vi "ELVIS III v1.0 AI Block Read.vi"(6 "AI FIFO Sample Rate":dbl=1000.0 min=1000.0 max=1000000.0, 7 "Scale Constants Array":T1, 8 "error in (no error)":errorcluster, 9 "Number of Samples":u32=1000, 10 "AI (N Samples) Channels List":T3, 11 "myRIO Ref In":T5) -> (0 "error out":errorcluster, 2 "dbl Scaled Value List":dbl[][](array[numeric]), 3 "myRIO Ref Out":T5)   [LabVIEW 2021]
uses:
  <vilib>/myRIO/Common/Instrument Driver Framework/Utilities/typedefs/myRIO v1.0 Reference.ctl
  <vilib>/myRIO/Common/Instrument Driver Framework/Utilities/typedefs/Generic FPGA Reference.ctl
  <vilib>/myRIO/Common/Instrument Driver Framework/myRIO v1.0/AI Block/typedefs/AI Block Channels List.ctl
  <vilib>/myRIO/Common/Instrument Driver Framework/myRIO v1.0/AI Block/typedefs/AI Block Channels Enum.ctl
  <vilib>/myRIO/Common/Instrument Driver Framework/Utilities/typedefs/Analog Scaling Constants List.ctl
  <vilib>/myRIO/Common/Instrument Driver Framework/Utilities/typedefs/Analog Scaling Constants.ctl
  <vilib>/myRIO/Common/Instrument Driver Framework/ELVIS III v1.0/AI Block/typedefs/ELVIS III AI Block Channels FPGA Reference.ctl
  <vilib>/myRIO/Common/Instrument Driver Framework/myRIO v1.0/Resource Manager/vis/myRIO v1.0 Block Write Configuration.vi
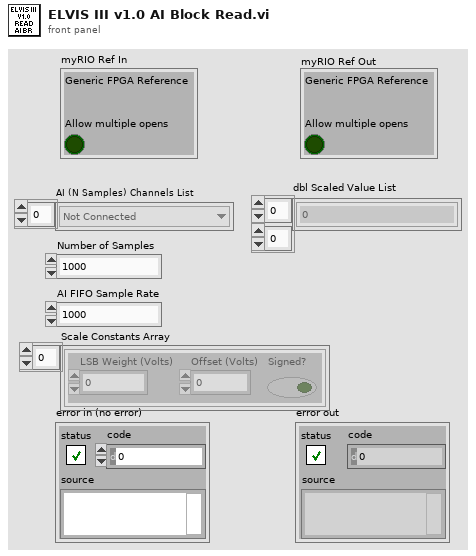
[diagram p1: front panel]
types:
  T1 = typedef "Analog Scaling Constants List.ctl" = T2[]
  T2 = typedef "Analog Scaling Constants.ctl" = cluster{"LSB Weight (Volts)":dbl, "Offset (Volts)":dbl, "Signed?":bool}
  T3 = typedef "AI Block Channels List.ctl" = T4[]
  T4 = typedef "AI Block Channels Enum.ctl" = enum16{"Not Connected", "A/AI0 (N Samples)", "A/AI1 (N Samples)", "A/AI2 (N Samples)", "A/AI3 (N Samples)", "A/AI4 (N Samples)", "A/AI5 (N Samples)", "A/AI6 (N Samples)", "A/AI7 (N Samples)", "A/AI0 (DIFF N Samples)", "A/AI1 (DIFF N Samples)", "A/AI2 (DIFF N Samples)", "A/AI3 (DIFF N Samples)", "B/AI0 (N Samples)", "B/AI1 (N Samples)", "B/AI2 (N Samples)", "B/AI3 (N Samples)", "B/AI4 (N Samples)", "B/AI5 (N Samples)", "B/AI6 (N Samples)", "B/AI7 (N Samples)", "B/AI0 (DIFF N Samples)", "B/AI1 (DIFF N Samples)", "B/AI2 (DIFF N Samples)", "B/AI3 (DIFF N Samples)"}
  T5 = typedef "myRIO v1.0 Reference.ctl" = cluster{"Generic FPGA Reference":T6, "Allow multiple opens":bool}
  T6 = typedef "Generic FPGA Reference.ctl" = refnum<k20>
  T7 = typedef "ELVIS III AI Block Channels FPGA Reference.ctl" = refnum<k20>
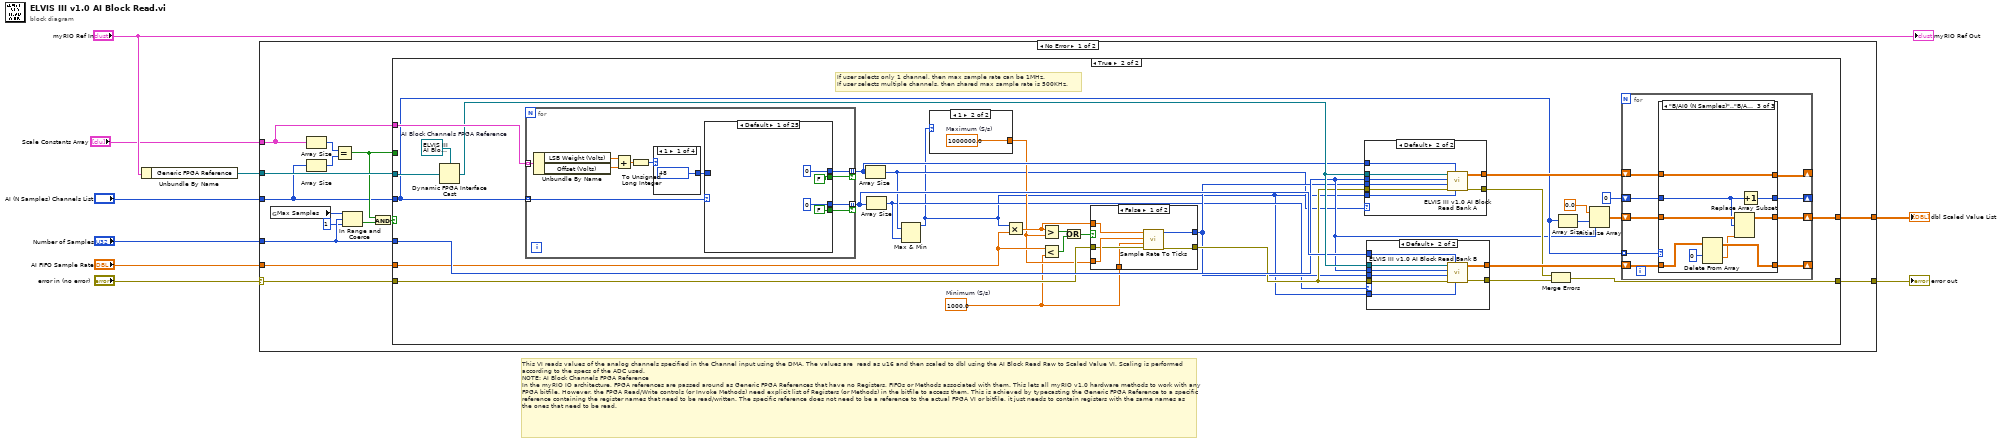
[diagram p0: block diagram]
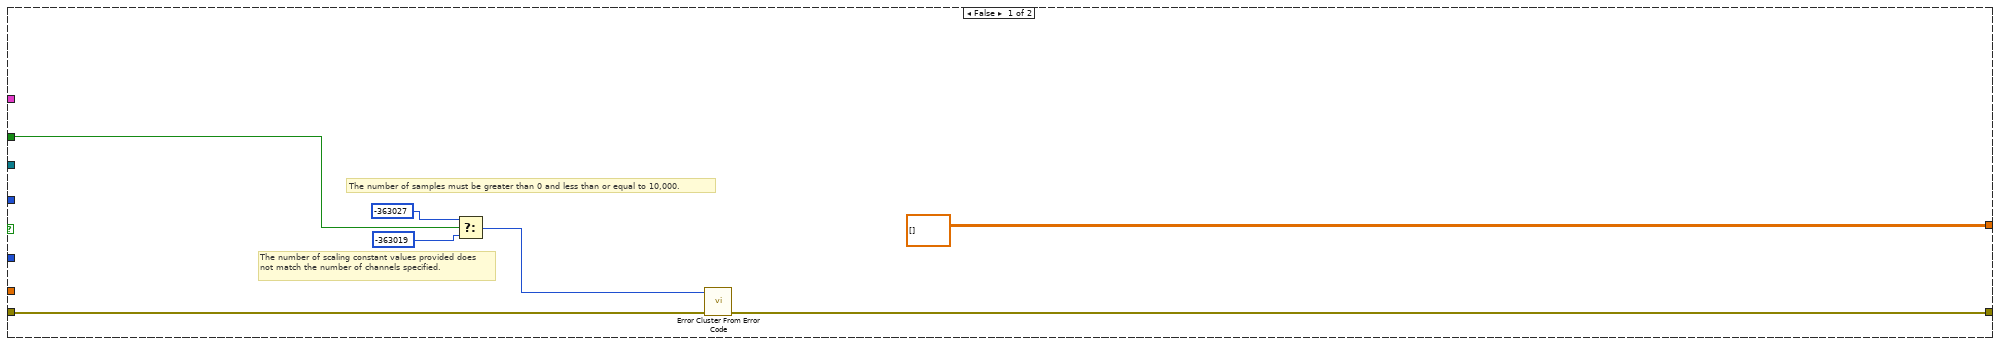
[diagram p2: hidden frame]
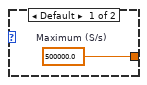
[diagram p3: hidden frame]
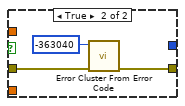
[diagram p4: hidden frame]
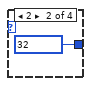
[diagram p5: hidden frame]
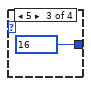
[diagram p6: hidden frame]
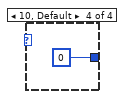
[diagram p7: hidden frame]
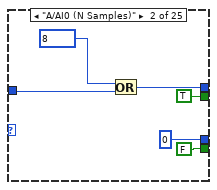
[diagram p8: hidden frame]
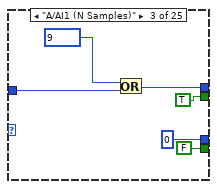
[diagram p9: hidden frame]
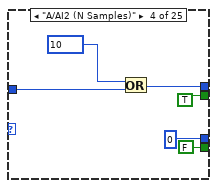
[diagram p10: hidden frame]
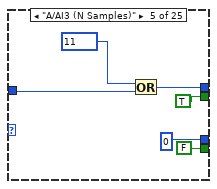
[diagram p11: hidden frame]
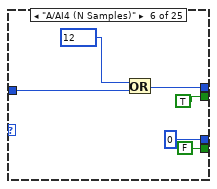
[diagram p12: hidden frame]
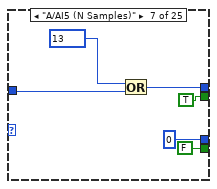
[diagram p13: hidden frame]
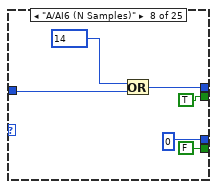
[diagram p14: hidden frame]
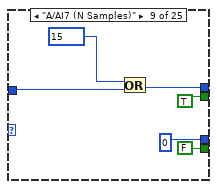
[diagram p15: hidden frame]
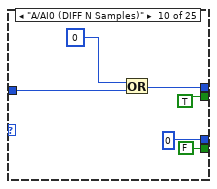
[diagram p16: hidden frame]
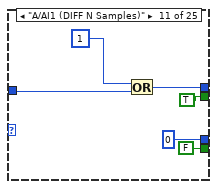
[diagram p17: hidden frame]
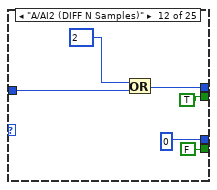
[diagram p18: hidden frame]
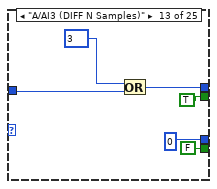
[diagram p19: hidden frame]
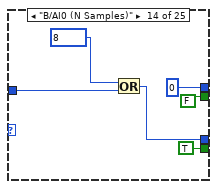
[diagram p20: hidden frame]
diagram:
  # "This VI reads values of the analog channels specified in the Channel input using the DMA. The values are  read as u16 and then scaled to dbl using the AI Block Read Raw to Scaled Value VI. Scaling is performed according to the specs of the ADC used.\nNOTE: AI Block Channels FPGA Reference\nIn the myRIO IO architecture, FPGA references are passed around as Generic FPGA References that have no Registers, FIFOs or Methods associated with them. This lets all myRIO v1.0 hardware methods to work with any FPGA bitfile. However, the FPGA Read/Write controls (or Invoke Methods) need explicit list of Registers (or Methods) in the bitfile to access them. This is achieved by typecasting the Generic FPGA Reference to a specific reference containing the register names that need to be read/written. The specific reference does not need to be a reference to the actual FPGA VI or bitfile, it just needs to contain registers with the same names as the ones that need to be read."
  n1 = Unbundle By Name("myRIO Ref In") -> ("Generic FPGA Reference"=w6:T6)
  n2 = case shown="No Error" "error in (no error)" {
    selector: "error in (no error)" -> [w10 w289]
    tunnel: w6 -> [w24 _]
    tunnel: [w23 w289] -> w9
    tunnel: [w22 dbl[][] [] ("dbl Scaled Value")] -> w8
    tunnel: "AI (N Samples) Channels List" -> [w12 _]
    tunnel: "AI FIFO Sample Rate" -> [w11 _]
    tunnel: "Number of Samples" -> [w16 _]
    tunnel: "Scale Constants Array" -> [w13 _]
    frame No Error {
      n3 = global read "myRIO v1.0 Block Write Configuration.vi" "Max Samples"() -> (w17:u32)
      n4 = Array Size(array=w13) -> (size(s)=w20:i32)
      n5 = Array Size(array=w12) -> (size(s)=w21:i32)
      n6 = Equal?(x=w20, y=w21) -> (x = y?=w18:bool)
      n7 = In Range and Coerce(upper limit=w17, x=w16, lower limit=u32 1) -> (In Range?=w14:bool)  [unwired: 1 out]
      n8 = And(x=w18, y=w14) -> (x .and. y?=w19:bool)
      n9 = case shown="True" w19 {
        tunnel: w24 -> [_ w61]
        tunnel: [w30 w55] -> w23
        tunnel: w10 -> [w31 w40]
        tunnel: [dbl[][] [] ("dbl Scaled Value") w58] -> w22
        tunnel: w16 -> [_ w47]
        tunnel: w12 -> [_ w50]
        tunnel: w18 -> [w28 _]
        tunnel: w13 -> [_ w54]
        tunnel: w11 -> [_ w42]
        frame False {
          # "The number of samples must be greater than 0 and less than or equal to 10,000."
          # "The number of scaling constant values provided does not match the number of channels specified."
          n10 = Select(t=-363027 ("error code (0)"), s=w28, f=-363019 ("error code (0)")) -> (s? t:f=w27:i32)
          n11 = call <vilib>:"Error Cluster From Error Code.vi"("error in (no error)"=w31, "error code (0)"=w27) -> ("error out"=w30:errorcluster)  [unwired: 7 in]
        }
        frame True {
          w35 = 1000.0  # Minimum (S/s)
          w62 = T7 refnum  # AI Block Channels FPGA Reference
          # "If user selects only 1 channel, then max sample rate can be 1MHz.\nIf user selects multiple channels, then shared max sample rate is 500KHz."
          n12 = Dynamic FPGA Interface Cast(Session In=w62, Type=w61) -> (Session Out=w53:T7)
          n13 = for {
            tunnel: w50 -> [w83] mode=indexing
            tunnel: w54 -> [w75] mode=indexing
            tunnel: [w84] -> w52 mode=indexing if=w82
            tunnel: [w81] -> w51 mode=indexing if=w80
            n14 = Unbundle By Name(w75) -> ("LSB Weight (Volts)"=w77:dbl, "Offset (Volts)"=w76:dbl)
            n15 = Add(x=w77, y=w76) -> (x+y=w78:dbl)
            n16 = To Unsigned Long Integer(number=w78) -> (unsigned 32bit integer=w79:u32)
            n17 = case shown="1" w79 {
              tunnel: [u8 48 u8 32 u8 16 u8 0] -> w74
              frame 1 {
              }
              frame 2 {
              }
              frame 5 {
              }
              frame 10, Default {
              }
            }
            n18 = case shown="Default" w83 {
              tunnel: [u8 0 w94 w100 w106 w112 w118 w124 w130 w136 w142 w148 w154 w160 u8 0 u8 0 u8 0 u8 0 u8 0 u8 0 u8 0 u8 0 u8 0 u8 0 u8 0 u8 0] -> w84
              tunnel: [FALSE TRUE TRUE TRUE TRUE TRUE TRUE TRUE TRUE TRUE TRUE TRUE TRUE FALSE FALSE FALSE FALSE FALSE FALSE FALSE FALSE FALSE FALSE FALSE FALSE] -> w82
              tunnel: [u8 0 u8 0 u8 0 u8 0 u8 0 u8 0 u8 0 u8 0 u8 0 u8 0 u8 0 u8 0 u8 0 w166 w172 w178 w184 w190 w196 w202 w208 w214 w220 w226 w232] -> w81
              tunnel: [FALSE FALSE FALSE FALSE FALSE FALSE FALSE FALSE FALSE FALSE FALSE FALSE FALSE TRUE TRUE TRUE TRUE TRUE TRUE TRUE TRUE TRUE TRUE TRUE TRUE] -> w80
              tunnel: w74 -> [_ w93 w99 w105 w111 w117 w123 w129 w135 w141 w147 w153 w159 w165 w171 w177 w183 w189 w195 w201 w207 w213 w219 w225 w231]
              frame Default {
              }
              frame "A/AI0 (N Samples)" {
                n19 = Or(x=u8 8, y=w93) -> (x .or. y?=w94:u8)
              }
              frame "A/AI1 (N Samples)" {
                n20 = Or(x=u8 9, y=w99) -> (x .or. y?=w100:u8)
              }
              frame "A/AI2 (N Samples)" {
                n21 = Or(x=u8 10, y=w105) -> (x .or. y?=w106:u8)
              }
              frame "A/AI3 (N Samples)" {
                n22 = Or(x=u8 11, y=w111) -> (x .or. y?=w112:u8)
              }
              frame "A/AI4 (N Samples)" {
                n23 = Or(x=u8 12, y=w117) -> (x .or. y?=w118:u8)
              }
              frame "A/AI5 (N Samples)" {
                n24 = Or(x=u8 13, y=w123) -> (x .or. y?=w124:u8)
              }
              frame "A/AI6 (N Samples)" {
                n25 = Or(x=u8 14, y=w129) -> (x .or. y?=w130:u8)
              }
              frame "A/AI7 (N Samples)" {
                n26 = Or(x=u8 15, y=w135) -> (x .or. y?=w136:u8)
              }
              frame "A/AI0 (DIFF N Samples)" {
                n27 = Or(x=u8 0, y=w141) -> (x .or. y?=w142:u8)
              }
              frame "A/AI1 (DIFF N Samples)" {
                n28 = Or(x=u8 1, y=w147) -> (x .or. y?=w148:u8)
              }
              frame "A/AI2 (DIFF N Samples)" {
                n29 = Or(x=u8 2, y=w153) -> (x .or. y?=w154:u8)
              }
              frame "A/AI3 (DIFF N Samples)" {
                n30 = Or(x=u8 3, y=w159) -> (x .or. y?=w160:u8)
              }
              frame "B/AI0 (N Samples)" {
                n31 = Or(x=u8 8, y=w165) -> (x .or. y?=w166:u8)
              }
              frame "B/AI1 (N Samples)" {
                n32 = Or(x=u8 9, y=w171) -> (x .or. y?=w172:u8)
              }
              frame "B/AI2 (N Samples)" {
                n33 = Or(x=u8 10, y=w177) -> (x .or. y?=w178:u8)
              }
              frame "B/AI3 (N Samples)" {
                n34 = Or(x=u8 11, y=w183) -> (x .or. y?=w184:u8)
              }
              frame "B/AI4 (N Samples)" {
                n35 = Or(x=u8 12, y=w189) -> (x .or. y?=w190:u8)
              }
              frame "B/AI5 (N Samples)" {
                n36 = Or(x=u8 13, y=w195) -> (x .or. y?=w196:u8)
              }
              frame "B/AI6 (N Samples)" {
                n37 = Or(x=u8 14, y=w201) -> (x .or. y?=w202:u8)
              }
              frame "B/AI7 (N Samples)" {
                n38 = Or(x=u8 15, y=w207) -> (x .or. y?=w208:u8)
              }
              frame "B/AI0 (DIFF N Samples)" {
                n39 = Or(x=u8 0, y=w213) -> (x .or. y?=w214:u8)
              }
              frame "B/AI1 (DIFF N Samples)" {
                n40 = Or(x=u8 1, y=w219) -> (x .or. y?=w220:u8)
              }
              frame "B/AI2 (DIFF N Samples)" {
                n41 = Or(x=u8 2, y=w225) -> (x .or. y?=w226:u8)
              }
              frame "B/AI3 (DIFF N Samples)" {
                n42 = Or(x=u8 3, y=w231) -> (x .or. y?=w232:u8)
              }
            }
          }
          n43 = Array Size(array=w52) -> (size(s)=w34:i32)
          n44 = Array Size(array=w51) -> (size(s)=w33:i32)
          n45 = Max & Min(x=w34, y=w33) -> (max(x,y)=w32:i32)  [unwired: 1 out]
          n46 = case shown="1" w32 {
            tunnel: [w63 w64] -> w36
            frame Default {
              w63 = 500000.0  # Maximum (S/s)
            }
            frame 1 {
              w64 = 1000000.0  # Maximum (S/s)
            }
          }
          n47 = Multiply(x=w32, y=w42) -> (x*y=w37:dbl)
          n48 = Greater?(x=w37, y=w36) -> (0:w44:bool)
          n49 = Less?(x=w42, y=w35) -> (x < y?=w43:bool)
          n50 = Or(x=w44, y=w43) -> (x .or. y?=w41:bool)
          n51 = case shown="False" w41 {
            tunnel: w40 -> [w67 w72]
            tunnel: [w70 w71] -> w39
            tunnel: [w65 _] -> w38
            tunnel: w37 -> [w69 _]
            tunnel: w36 -> [w68 _]
            tunnel: w35 -> [w66 _]
            frame False {
              n52 = call <vilib>:"Sample Rate To Ticks.vi"("error in (no error)"=w67, "Minimum (S/s)"=w66, "Maximum (S/s)"=w68, "Sample Rate (S/s)"=w69) -> ("error out"=w70:errorcluster, "Count (tick/s)"=w65:u32)  [unwired: 5 in, 1 out]
            }
            frame True {
              n53 = call <vilib>:"Error Cluster From Error Code.vi"("error in (no error)"=w72, "error code (0)"=-363040) -> ("error out"=w71:errorcluster)  [unwired: 7 in]
            }
          }
          n54 = case shown="Default" w34 {
            tunnel: w53 -> [_ w287]
            tunnel: w47 -> [_ w286]
            tunnel: w38 -> [_ w285]
            tunnel: [dbl[][] [] ("Data") w284] -> w60
            tunnel: w39 -> [w278 w283]
            tunnel: [w278 w282] -> w57
            tunnel: w52 -> [_ w281]
            tunnel: w32 -> [_ w280]
            frame 0 {
            }
            frame Default {
              n55 = call <vilib>:"ELVIS III v1.0 AI Block Read Bank A.vi"("CNT"=w280, "Bank Config"=w281, "error in (no error)"=w283, "Count (tick/s)"=w285, "Number of Samples"=w286, "AI Block Channels FPGA Reference"=w287) -> ("error out"=w282:errorcluster, "Data"=w284:dbl[][])  [unwired: 4 in]
            }
          }
          n56 = case shown="Default" w33 {
            tunnel: w53 -> [_ w246]
            tunnel: w47 -> [_ w245]
            tunnel: w38 -> [_ w244]
            tunnel: [dbl[][] [] ("Data") w243] -> w59
            tunnel: w39 -> [w237 w242]
            tunnel: [w237 w241] -> w56
            tunnel: w51 -> [_ w240]
            tunnel: w32 -> [_ w239]
            frame 0 {
            }
            frame Default {
              n57 = call <vilib>:"ELVIS III v1.0 AI Block Read Bank B.vi"("CNT"=w239, "Bank Config"=w240, "error in (no error)"=w242, "Count (tick/s)"=w244, "Number of Samples"=w245, "AI Block Channels FPGA Reference"=w246) -> ("error out"=w241:errorcluster, "Data"=w243:dbl[][])  [unwired: 4 in]
            }
          }
          n58 = Merge Errors(w57, w56) -> (w55:errorcluster)
          n59 = Array Size(array=w50) -> (size(s)=w49:i32)
          n60 = Initialize Array(0.0, w49, w47) -> (w45:dbl[][])
          n61 = for {
            tunnel: w50 -> [w255] mode=indexing
            shift-right: [w252] -> _
            shift-left: w60 -> [w254]
            shift-right: [w247] -> w58
            shift-left: w45 -> [w250]
            shift-right: [w251] -> _
            shift-left: w59 -> [w253]
            shift-right: [w248] -> _
            shift-left: 0 -> [w249]
            n62 = case shown="\"B/AI0 (N Samples)\"..\"B/AI3 (DIFF N Samples)\"" w255 {
              tunnel: w254 -> [w259 w268 w275]
              tunnel: [w259 w266 w275] -> w252
              tunnel: w253 -> [w258 w265 w276]
              tunnel: [w258 w265 w274] -> w251
              tunnel: w250 -> [w256 w263 w273]
              tunnel: w249 -> [w257 w262 w270]
              tunnel: [w257 w261 w269] -> w248
              tunnel: [w256 w260 w272] -> w247
              frame "Not Connected", Default {
              }
              frame "A/AI0 (N Samples)".."A/AI3 (DIFF N Samples)" {
                n63 = Delete From Array(array=w268, index (row)=0) -> (deleted portion=w264:dbl[], array with subset deleted=w266:dbl[][])  [unwired: 2 in]
                n64 = Replace Array Subset(array=w263, new element=w264, index (row)=w262) -> (w260:dbl[][])  [unwired: 1 in]
                n65 = Increment(x=w262) -> (x+1=w261:i32)
              }
              frame "B/AI0 (N Samples)".."B/AI3 (DIFF N Samples)" {
                n66 = Delete From Array(array=w276, index (row)=0) -> (deleted portion=w271:dbl[], array with subset deleted=w274:dbl[][])  [unwired: 2 in]
                n67 = Replace Array Subset(array=w273, new element=w271, index (row)=w270) -> (w272:dbl[][])  [unwired: 1 in]
                n68 = Increment(x=w270) -> (x+1=w269:i32)
              }
            }
          }
        }
      }
    }
    frame Error {
      # "There is an incoming error so there it nothing to do."
    }
  }
  "error out" <- w9
  "dbl Scaled Value List" <- w8
  "myRIO Ref Out" <- "myRIO Ref In"
